vi "Sqlite Query.vi"(0 "DB Path":string, 1 "SQL Query":string, 5 "Include RowID":bool, 7 "Tables Name":string, 11 "error in (no error)":errorcluster) -> (3 "Results":string[][](array[string]), 4 "DB Path Out":string, 15 "error out":errorcluster)   [LabVIEW 2016]
uses:
  <vilib>/LabVIEW Open Source Project/OpenSerializer.Base64/Base64_ByteLUT.vi
  <userlib>/_LVST/sqlite_api/Core/Query/SQLite_Query-Standard.vi
  <userlib>/_LVST/sqlite_api/Core/Tables/SQLite_List Columns.vi
  <vilib>/LabVIEW Open Source Project/OpenSerializer.Base64/Serializer.Base64.lvclass
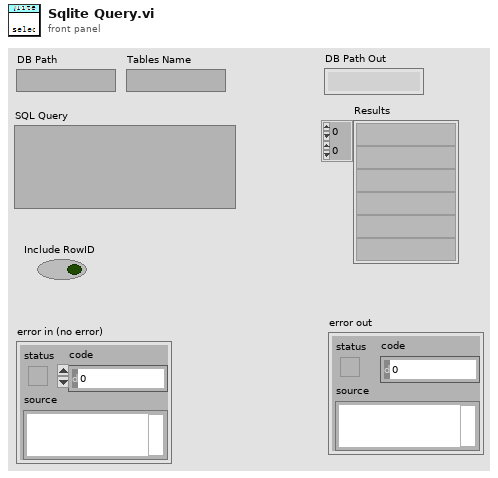
[diagram p1: front panel]
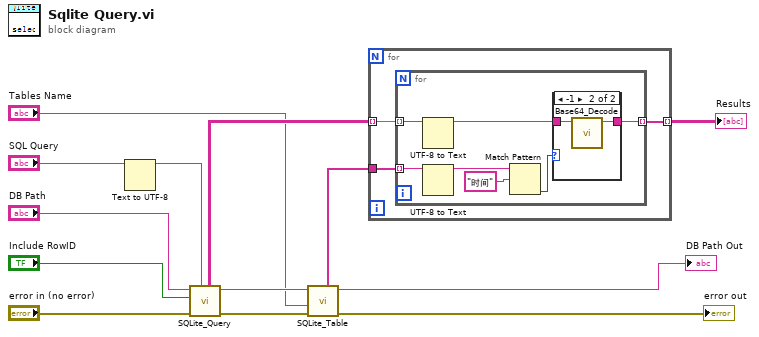
[diagram p0: block diagram]
diagram:
  n1 = Text to UTF-8(11:"SQL Query") -> (3:w8:string)  [unwired: 2 in, 1 out]
  n2 = call-poly <userlib>:"SQLite_Query.vi"("SQL Query"=w8, "error in (no error)"="error in (no error)", "Include RowID"="Include RowID", "DB Path"="DB Path") -> ("error out"=w4:errorcluster, "DB Path Out"=w6:string, "Results"=w7:string[][])  [unwired: 2 in, 1 out]
  n3 = call-poly <userlib>:"SQLite_Table.vi"("DB Path"=w6, "Table Name"="Tables Name", "error in (no error)"=w4) -> ("Columns"=w1:string[], "DB Path Out"=→"DB Path Out":string, "error out"=→"error out":errorcluster)  [unwired: 4 in, 1 out]
  n4 = for {
    tunnel: w7 -> [w16] mode=indexing
    tunnel: [w15] -> w13 mode=indexing
    tunnel: w1 -> [w14]
    n5 = for {
      tunnel: w16 -> [w18] mode=indexing
      tunnel: [w17] -> w15 mode=indexing
      tunnel: w14 -> [w19] mode=indexing
      n6 = UTF-8 to Text(11:w18) -> (3:w20:string)  [unwired: 2 in, 1 out]
      n7 = UTF-8 to Text(11:w19) -> (3:w21:string)  [unwired: 2 in, 1 out]
      n8 = Match Pattern(string=w21, regular expression="时间" ("正则表达式")) -> (offset past match=w22:i32)  [unwired: 1 in, 3 out]
      n9 = case shown="-1" w22 {
        tunnel: w20 -> [w24 w26]
        tunnel: [w24 w25] -> w17
        frame 0, Default {
        }
        frame -1 {
          n10 = call <vilib>:"Base64_Decode.vi"("Base64 String"=w26) -> ("Decoded String"=w25:string)  [unwired: 9 in, 1 out]
        }
      }
    }
  }
  "Results" <- w13
